vi "Update Palette.vi"() -> ()   [LabVIEW 2023]
doc: "Illustrates how to use the Read Palette.vi and Write Palette.vi to make a change to an existing palette."
uses:
  <vilib>/Palette API/Palette Menu/Public Type Define/Palette type.ctl
  <vilib>/Palette API/Palette Menu/Palette Menu.lvlib
panel:
  in  "New Display Name":string="Palette API Evaluation"
  # "Overview: Demonstrates the use of the Palette Editing VIs to update an existing palette configuration.\nInstructions:\n1. Make sure you have already run the Create New Palette.vi example.\n2. Run this VI. It will change the display name of the Functions > User Libraries > Palette API subpalette. See the block diagram for more information."
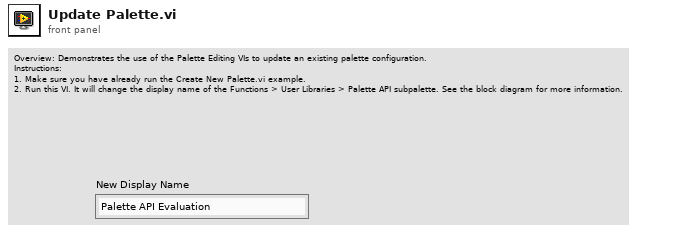
[diagram p1: front panel]
types:
  T1 = typedef "Palette Menu.lvlib/Palette type.ctl" = i32
  T2 = typedef "Palette Menu.lvlib/Palette Data.ctl" = cluster{"display name":string, "view format":T3, "palette width":i16, "items":T4, "256 color icon":picture, "B&W color icon":picture, "help information":T6, "palette description":string, "synchronize information":T7}
  T3 = typedef "Palette Menu.lvlib/View Format.ctl" = u16
  T4 = typedef "Palette Menu.lvlib/Items.ctl" = T5[]
  T5 = typedef "Palette Menu.lvlib/Item.ctl" = cluster{"item path":path, "library path":path, "use default lvlib palette":bool, "short name":string, "place VI contents":bool, "hide synchronized item":bool, "reserve spot for synch item":bool, "configure when placing VI contents":bool}
  T6 = typedef "Palette Menu.lvlib/Help Info.ctl" = cluster{"help tag":string, "help file path ":path}
  T7 = typedef "Palette Menu.lvlib/Synchronize Info.ctl" = cluster{"synchronize with directory":bool, "synchronize directory path":path}
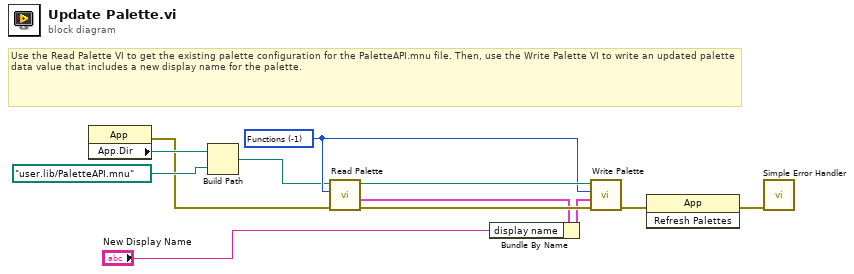
[diagram p0: block diagram]
diagram:
  w6 = T1 -1 items=["Functions"=-1, "Controls"=-2] ("palette type")
  # "Use the Read Palette VI to get the existing palette configuration for the PaletteAPI.mnu file. Then, use the Write Palette VI to write an updated palette data value that includes a new display name for the palette."
  n1 = property class="App"() -> (error out=w1:errorcluster, "App.Dir"=w5:path)  [unwired: 2 in, 1 out]
  n2 = Build Path(base path=w5, name or relative path=path "user.lib/PaletteAPI.mnu") -> (appended path=w3:path)
  n3 = call <vilib>:"Read Palette.vi"("error in (no error)"=w1, "palette type"=w6, "palette path"=w3) -> ("error out"=w12:errorcluster, "palette data"=w11:T2, "duplicate palette path"=w9:path)  [unwired: 1 in, 5 out]
  n4 = Bundle By Name(cluster=w11, "display name"="New Display Name") -> (w10:T2)
  n5 = call <vilib>:"Write Palette.vi"("error in (no error)"=w12, "palette data"=w10, "palette type"=w6, "palette path"=w9) -> ("error out"=w7:errorcluster)  [unwired: 1 in, 6 out]
  n6 = invoke class="App" method="Refresh Palettes"(error in=w7) -> (error out=w8:errorcluster)  [unwired: 2 in, 2 out]
  n7 = call <vilib>:"Simple Error Handler.vi"("error in (no error)"=w8) -> ()  [unwired: 1 in, 8 out]
